vi "F_F1_F2.vi"(6 "计算参数 in":T2, 7 "输入参数":T1, 8 "进油口压力数组 in":dbl[](array[numeric])) -> (0 "计算参数 out":T2, 1 "输入参数 out":T1, 2 "进油口压力数组 out":dbl[](array[numeric]))   [LabVIEW 2013]
doc: "此程序计算开启关闭时间\nCL=tv2-tv1\nOP=ts2-ts1"
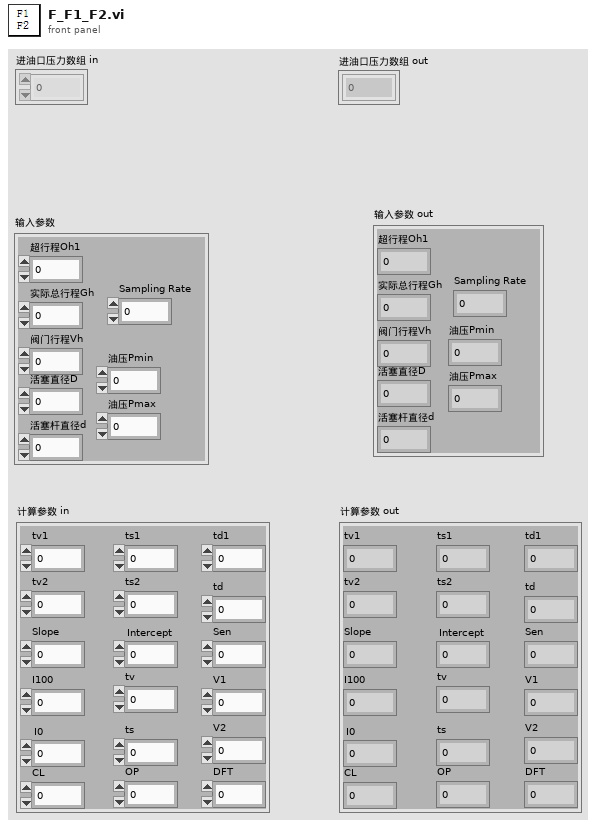
[diagram p1: front panel]
types:
  T1 = cluster{"超行程Oh1":dbl, "实际总行程Gh":dbl, "阀门行程Vh":dbl, "活塞直径D":dbl, "活塞杆直径d":dbl, "油压Pmin":dbl, "油压Pmax":dbl, "Sampling Rate":dbl}
  T2 = cluster{"tv1":dbl, "tv2":dbl, "tv":dbl, "ts1":dbl, "ts2":dbl, "ts":dbl, "td1":dbl, "td":dbl, "Slope":dbl, "Intercept":dbl, "I100":dbl, "I0":dbl, "Sen":dbl, "V1":dbl, "V2":dbl, "CL":dbl, "OP":dbl, "DFT":dbl}
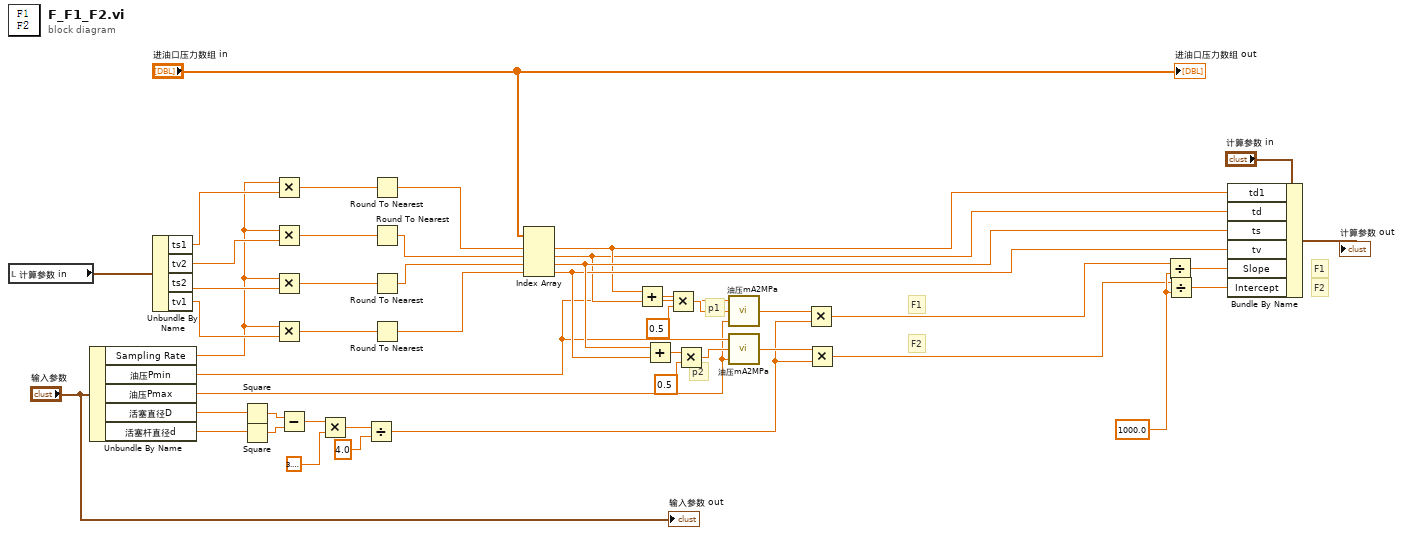
[diagram p0: block diagram]
diagram:
  w18 = 1000.0
  # "F2"
  # "F1"
  # "F2"
  # "F1"
  # "p2"
  # "p1"
  n1 = local read "计算参数 in"() -> (w44:T2)
  n2 = Unbundle By Name("输入参数") -> ("Sampling Rate"=w1:dbl, "油压Pmin"=w3:dbl, "油压Pmax"=w2:dbl, "活塞直径D"=w31:dbl, "活塞杆直径d"=w30:dbl)
  n3 = Unbundle By Name(w44) -> ("ts1"=w43:dbl, "tv2"=w42:dbl, "ts2"=w41:dbl, "tv1"=w40:dbl)
  n4 = Square(x=w31) -> (x^2=w29:dbl)
  n5 = Square(x=w30) -> (x^2=w28:dbl)
  n6 = Multiply(x=w1, y=w43) -> (x*y=w38:dbl)
  n7 = Multiply(x=w1, y=w42) -> (x*y=w39:dbl)
  n8 = Multiply(x=w1, y=w41) -> (x*y=w37:dbl)
  n9 = Multiply(x=w1, y=w40) -> (x*y=w36:dbl)
  n10 = Subtract(x=w29, y=w28) -> (x-y=w27:dbl)
  n11 = Multiply(x=w27, y=3.141592653589793) -> (x*y=w25:dbl)
  n12 = Divide(x=w25, y=4.0) -> (x/y=w20:dbl)
  n13 = Round To Nearest(number=w38) -> (nearest integer value=w35:dbl)
  n14 = Round To Nearest(number=w39) -> (nearest integer value=w34:dbl)
  n15 = Round To Nearest(number=w37) -> (nearest integer value=w33:dbl)
  n16 = Round To Nearest(number=w36) -> (nearest integer value=w32:dbl)
  n17 = Index Array(array="进油口压力数组 in", index #1=w35, index #2=w34, index #3=w33, index #4=w32) -> (element #1=w6:dbl, element #2=w5:dbl, element #3=w14:dbl, element #4=w13:dbl)
  n18 = Add(x=w6, y=w5) -> (x+y=w9:dbl)
  n19 = Add(x=w14, y=w13) -> (x+y=w12:dbl)
  n20 = Multiply(x=w9, y=0.5) -> (x*y=w7:dbl)
  n21 = Multiply(x=w12, y=0.5) -> (x*y=w10:dbl)
  n22 = call "油压mA2MPa.vi"("油压Max"=w2, "油压mA"=w7, "油压Min"=w3) -> ("油压MPa"=w22:dbl)  [unwired: 2 in]
  n23 = call "油压mA2MPa.vi"("油压Max"=w2, "油压mA"=w10, "油压Min"=w3) -> ("油压MPa"=w21:dbl)  [unwired: 2 in]
  n24 = Multiply(x=w22, y=w20) -> (x*y=w19:dbl)
  n25 = Multiply(x=w21, y=w20) -> (x*y=w16:dbl)
  n26 = Divide(x=w19, y=w18) -> (x/y=w17:dbl)
  n27 = Divide(x=w16, y=w18) -> (x/y=w15:dbl)
  n28 = Bundle By Name(cluster="计算参数 in", "td1"=w6, "td"=w5, "ts"=w14, "tv"=w13, "Slope"=w17, "Intercept"=w15) -> (→"计算参数 out":T2)
  "进油口压力数组 out" <- "进油口压力数组 in"
  "输入参数 out" <- "输入参数"
